vi "Read Cell Laser Diode Signal.vi"(8 "error in":errorcluster, 11 "PAS Data in":refnum<class "PAS Data.lvclass">) -> (0 "error out":errorcluster, 2 "lasDiodeData":waveform(i16), 3 "PAS Data out":refnum<class "PAS Data.lvclass">)   [LabVIEW 2014, in "PAS Library.lvlib" / "PAS Data.lvclass"]
uses:
  PAS Data.lvclass
  PAS Data.lvclass/PAS Data.ctl
  Cell/PAS Cell Data.lvclass
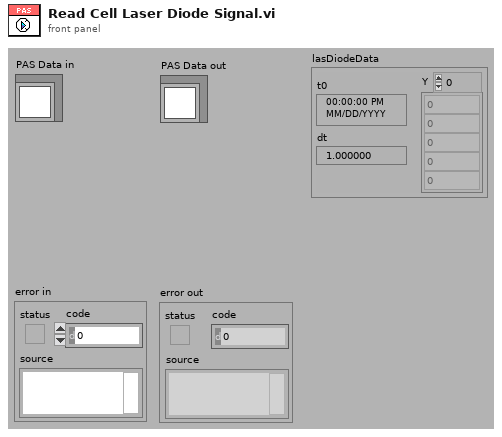
[diagram p1: front panel]
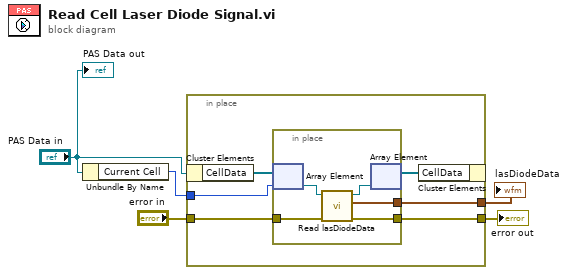
[diagram p0: block diagram]
diagram:
  n1 = Unbundle By Name("PAS Data in") -> ("Current Cell"=w4:i32)
  n2 = in-place {
    in-place-border: w4 -> [w11]
    in-place-border: "error in" -> [w10]
    in-place-border: [w9] -> w2
    in-place-border: [w6] -> w1
    n3 = in-place-cluster #1("PAS Data in") -> ("CellData"=w8:refnum<class "PAS Cell Data.lvclass">[])
    n4 = in-place {
      in-place-border: w10 -> [w15]
      in-place-border: [w13] -> w9
      in-place-border: [w12] -> w6
      n5 = in-place-array #2(w8, w11) -> (w16:refnum<class "PAS Cell Data.lvclass">)
      n6 = call "Read lasDiodeData.vi"("error in (no error)"=w15, "PAS Cell Data in"=w16) -> ("error out"=w13:errorcluster, "lasDiodeData"=w12:waveform(i16), "PAS Cell Data out"=w14:refnum<class "PAS Cell Data.lvclass">)  [unwired: 7 in]
      n7 = in-place-array #2(w14) -> (w7:refnum<class "PAS Cell Data.lvclass">[])  [unwired: 1 out]
    }
    n8 = in-place-cluster #1("CellData"=w7) -> ()  [unwired: 1 out]
  }
  "error out" <- w2
  "lasDiodeData" <- w1
  "PAS Data out" <- "PAS Data in"
